vi "Image Rotation Example.vi"() -> ()   [LabVIEW 2020]
doc: "G-Image example demonstrating image loading, rotation, and display."
uses:
  Image IO/Polymorphic VIs/Load Image (Path).vi
  G-Image.lvlib
panel:
  in  "Stop":bool
  out "2D Picture":picture
  in  "Filter":bool
  in  "Rotation (Degrees)":dbl(slide) step=1.0 scale=180.0..-180.0
  # "Instructions:\n1. Run the VI.\n2. Rotate the image using the slider.\n3. Toggle the Enable Filtering checkbox to compare unfiltered and filtered rotation image quality."
  # "G"
  # "-Image"
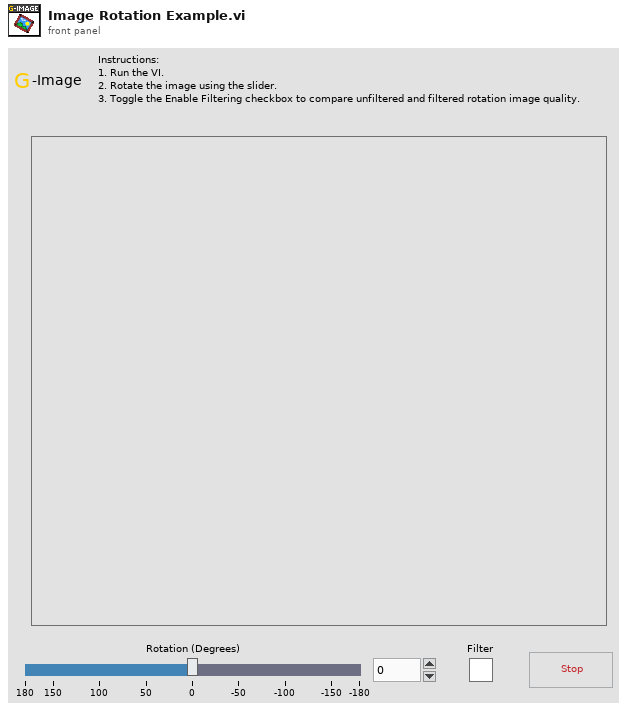
[diagram p1: front panel]
types:
  T1 = typedef "imagedata.ctl" = cluster{"image type":i32, "image depth":i32, "image":u8[], "mask":u8[], "colors":u32[], "Rectangle":cluster{"left":i16, "top":i16, "right":i16, "bottom":i16}}
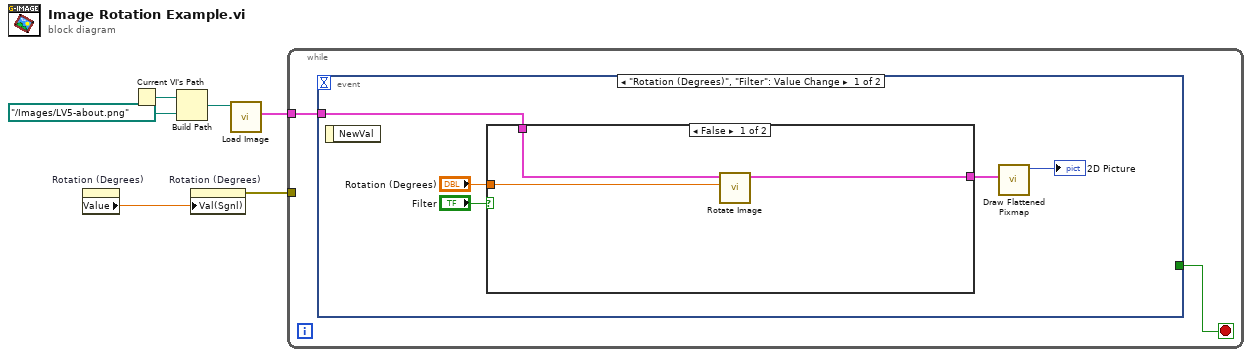
[diagram p0: block diagram]
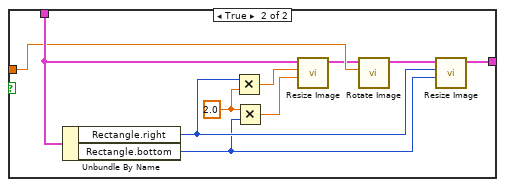
[diagram p2: hidden frame]
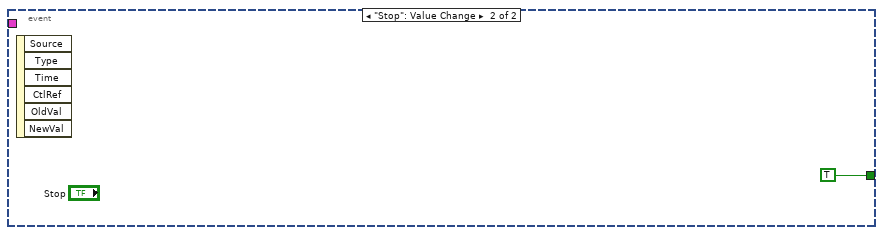
[diagram p3: hidden frame]
diagram:
  n1 = property on="Rotation (Degrees)" class="Slide (strict)"() -> ("Value"=w6:dbl)  [unwired: 2 in, 2 out]
  n2 = Current VI's Path() -> (path=w4:path)
  n3 = Build Path(base path=w4, name or relative path=path "../Images/LV5-about.png") -> (appended path=w2:path)
  n4 = property on="Rotation (Degrees)" class="Slide (strict)"("Val(Sgnl)"=w6) -> (error out=w5:errorcluster)  [unwired: 2 in, 1 out]
  n5 = call-poly "Load Image.vi"("Path In"=w2) -> ("Image"=w1:T1)  [unwired: 8 in, 2 out]
  n6 = while {
    tunnel: w1 -> [w8]
    tunnel: w5 -> [_]
    stop <- w7 stop-if-true
    n7 = event shown="[0] \"Rotation (Degrees)\", \"Filter\": Value Change" {
      selector: _ -> [_ _]
      dyn-events: _ -> [_ _]
      timeout: _ -> [_ _]
      tunnel: w8 -> [w13 _]
      tunnel: [_ TRUE] -> w7
      event "Rotation (Degrees)", "Filter": Value Change {
        n8 = event-data() -> ()  [unwired: 1 in, 1 out]
        n9 = case shown="False" "Filter" {
          tunnel: w13 -> [w15 w24]
          tunnel: "Rotation (Degrees)" -> [w16 w20]
          tunnel: [w14 w19] -> w9
          frame False {
            n10 = call "Rotate Image.vi"("Degrees"=w16, "Image"=w15) -> ("Rotated Image"=w14:T1)  [unwired: 8 in, 1 out]
          }
          frame True {
            w21 = 2.0 ("y")
            n11 = Unbundle By Name(w24) -> ("Rectangle.right"=w26:i16, "Rectangle.bottom"=w25:i16)
            n12 = Multiply(x=w26, y=w21) -> (x*y=w23:dbl)
            n13 = Multiply(x=w21, y=w25) -> (x*y=w22:dbl)
            n14 = call "Resize Image.vi"("Height"=w22, "Width"=w23, "Image"=w24) -> ("Resized Image"=w17:T1)  [unwired: 7 in, 1 out]
            n15 = call "Rotate Image.vi"("Degrees"=w20, "Image"=w17) -> ("Rotated Image"=w18:T1)  [unwired: 8 in, 1 out]
            n16 = call "Resize Image.vi"("Height"=w25, "Width"=w26, "Image"=w18) -> ("Resized Image"=w19:T1)  [unwired: 7 in, 1 out]
          }
        }
        n17 = call <vilib>:"Draw Flattened Pixmap.vi"("image data"=w9) -> ("new picture"=→"2D Picture":picture)  [unwired: 8 in]
      }
      event "Stop": Value Change {
        n18 = event-data() -> ()  [unwired: 1 in, 6 out]
      }
    }
  }
